vi "Add Comma.vi"(10 "Previous String":string, 11 "format string in":string) -> (3 "format string out":string)   [LabVIEW 2016, in "XControl Custom Time Display.xctl"]
uses:
  XControl Custom Time Display.xctl
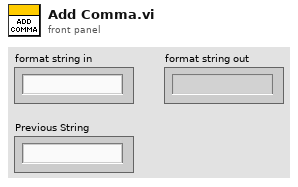
[diagram p1: front panel]
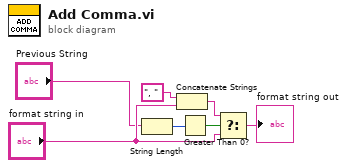
[diagram p0: block diagram]
diagram:
  n1 = String Length(string="Previous String") -> (length=w2:i32)
  n2 = Concatenate Strings(", ", "format string in") -> (w6:string)
  n3 = Greater Than 0?(x=w2) -> (x > 0?=w3:bool)
  n4 = Select(t=w6, s=w3, f="format string in") -> (s? t:f=→"format string out":string)
